vi "nanocal -- nuclear schottky fit -- 2x2 -- V9.vi"() -> ()   [LabVIEW 2021] (continued)
τ1\" -> 0.000000000000   ,  \"τS\" -> 0.000000000000   ,  \"τN\" -> 0.000000000000   ,  \"τC\" -> 0.000000000000   ,  \"κ0\" -> 0.000000000000   ,  \"mm1\" -> 0.000000000000   ,  \"mm2\" -> 0.000000000000   ,  \"mm3\" -> 0.000000000000   ,  \"T\" -> 0.300000000000   ,  \"B\" -> 10.000000000000   ,  \"θ\" -> 90.000000000000   ,  \"Reoff\" -> 0.000000000000   ,  \"Imoff\" -> 0.000000000000   ,  \"στ1\" -> 0.000000000000   ,  \"στS\" -> 0.000000000000   ,  \"στN\" -> 0.000000000000    |>   , \n\"IDS0630_220611_RAW_cal__ref_\" ->   <|    \"ζ\" -> 0.079968077159   ,  \"τ1\" -> 0.028703647271   ,  \"τS\" -> 0.027787521037   ,  \"τN\" -> 0.007458471541   ,  \"τC\" -> 0.001227018439   ,  \"κ0\" -> 0.000000002002   ,  \"mm1\" -> 0.000087530349   ,  \"mm2\" -> 0.017868351082   ,  \"mm3\" -> 0.050039331111   ,  \"T\" -> 0.360000000000   ,  \"B\" -> 10.000000000000   ,  \"θ\" -> 90.000000000000   ,  \"Reoff\" -> -6897959.183673471220   ,  \"Imoff\" -> 0.000000000000   ,  \"στ1\" -> 0.003375898444   ,  \"στS\" -> 0.000219600830   ,  \"στN\" -> 0.000437287365    |>   , \n\"IDS0630_220611_RAW_cal__sam_\" ->   <|    \"ζ\" -> 0.000000000000   ,  \"τ1\" -> 0.000000000000   ,  \"τS\" -> 0.000000000000   ,  \"τN\" -> 0.000000000000   ,  \"τC\" -> 0.000000000000   ,  \"κ0\" -> 0.000000000000   ,  \"mm1\" -> 0.000000000000   ,  \"mm2\" -> 0.000000000000   ,  \"mm3\" -> 0.000000000000   ,  \"T\" -> 0.360000000000   ,  \"B\" -> 10.000000000000   ,  \"θ\" -> 90.000000000000   ,  \"Reoff\" -> 0.000000000000   ,  \"Imoff\" -> 0.000000000000   ,  \"στ1\" -> 0.000000000000   ,  \"στS\" -> 0.000000000000   ,  \"στN\" -> 0.000000000000    |>   , \n\"IDS0631_220611_RAW_cal__ref_\" ->   <|    \"ζ\" -> 0.058778460979   ,  \"τ1\" -> 0.022115004364   ,  \"τS\" -> 0.025871969436   ,  \"τN\" -> 0.004788101555   ,  \"τC\" -> 0.001625064800   ,  \"κ0\" -> 0.000000002412   ,  \"mm1\" -> 0.000085411879   ,  \"mm2\" -> 0.015917070637   ,  \"mm3\" -> 0.040199809426   ,  \"T\" -> 0.420000000000   ,  \"B\" -> 10.000000000000   ,  \"θ\" -> 90.000000000000   ,  \"Reoff\" -> -2816326.530612244270   ,  \"Imoff\" -> 0.000000000000   ,  \"στ1\" -> 0.000587796710   ,  \"στS\" -> 0.000091605589   ,  \"στN\" -> 0.000126012019    |>   , \n\"IDS0631_220611_RAW_cal__sam_\" ->   <|    \"ζ\" -> 0.000000000000   ,  \"τ1\" -> 0.000000000000   ,  \"τS\" -> 0.000000000000   ,  \"τN\" -> 0.000000000000   ,  \"τC\" -> 0.000000000000   ,  \"κ0\" -> 0.000000000000   ,  \"mm1\" -> 0.000000000000   ,  \"mm2\" -> 0.000000000000   ,  \"mm3\" -> 0.000000000000   ,  \"T\" -> 0.420000000000   ,  \"B\" -> 10.000000000000   ,  \"θ\" -> 90.000000000000   ,  \"Reoff\" -> 0.000000000000   ,  \"Imoff\" -> 0.000000000000   ,  \"στ1\" -> 0.000000000000   ,  \"στS\" -> 0.000000000000   ,  \"στN\" -> 0.000000000000    |>   , \n\"IDS0632_220611_RAW_cal__ref_\" ->   <|    \"ζ\" -> 0.043876208110   ,  \"τ1\" -> 0.021478355659   ,  \"τS\" -> 0.024271049020   ,  \"τN\" -> 0.002270431826   ,  \"τC\" -> 0.001878964186   ,  \"κ0\" -> 0.000000003102   ,  \"mm1\" -> 0.000073722080   ,  \"mm2\" -> 0.017307979811   ,  \"mm3\" -> 0.033681638338   ,  \"T\" -> 0.520000000000   ,  \"B\" -> 10.000000000000   ,  \"θ\" -> 90.000000000000   ,  \"Reoff\" -> -1918367.346938774920   ,  \"Imoff\" -> 0.000000000000   ,  \"στ1\" -> 0.003137180042   ,  \"στS\" -> 0.000114620716   ,  \"στN\" -> 0.000177904413    |>   , \n\"IDS0632_220611_RAW_cal__sam_\" ->   <|    \"ζ\" -> 0.000000000000   ,  \"τ1\" -> 0.000000000000   ,  \"τS\" -> 0.000000000000   ,  \"τN\" -> 0.000000000000   ,  \"τC\" -> 0.000000000000   ,  \"κ0\" -> 0.000000000000   ,  \"mm1\" -> 0.000000000000   ,  \"mm2\" -> 0.000000000000   ,  \"mm3\" -> 0.000000000000   ,  \"T\" -> 0.520000000000   ,  \"B\" -> 10.000000000000   ,  \"θ\" -> 90.000000000000   ,  \"Reoff\" -> 0.000000000000   ,  \"Imoff\" -> 0.000000000000   ,  \"στ1\" -> 0.000000000000   ,  \"στS\" -> 0.000000000000   ,  \"στN\" -> 0.000000000000    |>   , \n\"IDS0633_220611_RAW_cal__ref_\" ->   <|    \"ζ\" -> 0.034677079160   ,  \"τ1\" -> 0.021718381386   ,  \"τS\" -> 0.023156430325   ,  \"τN\" -> 0.001263823282   ,  \"τC\" -> 0.002065959541   ,  \"κ0\" -> 0.000000003789   ,  \"mm1\" -> 0.000063900017   ,  \"mm2\" -> 0.018485786163   ,  \"mm3\" -> 0.030501731422   ,  \"T\" -> 0.620000000000   ,  \"B\" -> 10.000000000000   ,  \"θ\" -> 90.000000000000   ,  \"Reoff\" -> -1265306.122448978950   ,  \"Imoff\" -> 0.000000000000   ,  \"στ1\" -> 0.002060583109   ,  \"στS\" -> 0.000081647328   ,  \"στN\" -> 0.000097316031    |>   , \n\"IDS0633_220611_RAW_cal__sam_\" ->   <|    \"ζ\" -> 0.000000000000   ,  \"τ1\" -> 0.000000000000   ,  \"τS\" -> 0.000000000000   ,  \"τN\" -> 0.000000000000   ,  \"τC\" -> 0.000000000000   ,  \"κ0\" -> 0.000000000000   ,  \"mm1\" -> 0.000000000000   ,  \"mm2\" -> 0.000000000000   ,  \"mm3\" -> 0.000000000000   ,  \"T\" -> 0.620000000000   ,  \"B\" -> 10.000000000000   ,  \"θ\" -> 90.000000000000   ,  \"Reoff\" -> 0.000000000000   ,  \"Imoff\" -> 0.000000000000   ,  \"στ1\" -> 0.000000000000   ,  \"στS\" -> 0.000000000000   ,  \"στN\" -> 0.000000000000    |>   , \n\"IDS0634_220612_RAW_cal__ref_\" ->   <|    \"ζ\" -> 0.027036169383   ,  \"τ1\" -> 0.021733696350   ,  \"τS\" -> 0.021135918538   ,  \"τN\" -> 0.000553307170   ,  \"τC\" -> 0.002271656254   ,  \"κ0\" -> 0.000000005164   ,  \"mm1\" -> 0.000054257381   ,  \"mm2\" -> 0.019338329094   ,  \"mm3\" -> 0.026888385418   ,  \"T\" -> 0.820000000000   ,  \"B\" -> 10.000000000000   ,  \"θ\" -> 90.000000000000   ,  \"Reoff\" -> -938775.510204080491   ,  \"Imoff\" -> 0.000000000000   ,  \"στ1\" -> 0.001360200971   ,  \"στS\" -> 0.000123877284   ,  \"στN\" -> 0.000020166019    |>   , \n\"IDS0634_220612_RAW_cal__sam_\" ->   <|    \"ζ\" -> 0.000000000000   ,  \"τ1\" -> 0.000000000000   ,  \"τS\" -> 0.000000000000   ,  \"τN\" -> 0.000000000000   ,  \"τC\" -> 0.000000000000   ,  \"κ0\" -> 0.000000000000   ,  \"mm1\" -> 0.000000000000   ,  \"mm2\" -> 0.000000000000   ,  \"mm3\" -> 0.000000000000   ,  \"T\" -> 0.820000000000   ,  \"B\" -> 10.000000000000   ,  \"θ\" -> 90.000000000000   ,  \"Reoff\" -> 0.000000000000   ,  \"Imoff\" -> 0.000000000000   ,  \"στ1\" -> 0.000000000000   ,  \"στS\" -> 0.000000000000   ,  \"στN\" -> 0.000000000000    |>   , \n\"IDS0635_220612_RAW_cal__ref_\" ->   <|    \"ζ\" -> 0.022890647572   ,  \"τ1\" -> 0.021599440333   ,  \"τS\" -> 0.018784843036   ,  \"τN\" -> 0.000235286917   ,  \"τC\" -> 0.002353311778   ,  \"κ0\" -> 0.000000007245   ,  \"mm1\" -> 0.000047019578   ,  \"mm2\" -> 0.019399476842   ,  \"mm3\" -> 0.023961768735   ,  \"T\" -> 1.120000000000   ,  \"B\" -> 10.000000000000   ,  \"θ\" -> 90.000000000000   ,  \"Reoff\" -> -775510.204081632196   ,  \"Imoff\" -> 0.000000000000   ,  \"στ1\" -> 0.004256477992   ,  \"στS\" -> 0.000144718396   ,  \"στN\" -> 0.000029208339    |>   , \n\"IDS0635_220612_RAW_cal__sam_\" ->   <|    \"ζ\" -> 0.000000000000   ,  \"τ1\" -> 0.000000000000   ,  \"τS\" -> 0.000000000000   ,  \"τN\" -> 0.000000000000   ,  \"τC\" -> 0.000000000000   ,  \"κ0\" -> 0.000000000000   ,  \"mm1\" -> 0.000000000000   ,  \"mm2\" -> 0.000000000000   ,  \"mm3\" -> 0.000000000000   ,  \"T\" -> 1.120000000000   ,  \"B\" -> 10.000000000000   ,  \"θ\" -> 90.000000000000   ,  \"Reoff\" -> 0.000000000000   ,  \"Imoff\" -> 0.000000000000   ,  \"στ1\" -> 0.000000000000   ,  \"στS\" -> 0.000000000000   ,  \"στN\" -> 0.000000000000    |>   , \n\"IDS0636_220612_RAW_cal__ref_\" ->   <|    \"ζ\" -> 0.017457751366   ,  \"τ1\" -> 0.021556950502   ,  \"τS\" -> 0.013950093477   ,  \"τN\" -> 0.000069572481   ,  \"τC\" -> 0.002888715109   ,  \"κ0\" -> 0.000000012635   ,  \"mm1\" -> 0.000041283144   ,  \"mm2\" -> 0.016791744848   ,  \"mm3\" -> 0.021877055420   ,  \"T\" -> 1.900000000000   ,  \"B\" -> 10.000000000000   ,  \"θ\" -> 90.000000000000   ,  \"Reoff\" -> -285714.285714285448   ,  \"Imoff\" -> 0.000000000000   ,  \"στ1\" -> 0.002815711957   ,  \"στS\" -> 0.000085308545   ,  \"στN\" -> 0.000003509861    |>   , \n\"IDS0636_220612_RAW_cal__sam_\" ->   <|    \"ζ\" -> 0.000000000000   ,  \"τ1\" -> 0.000000000000   ,  \"τS\" -> 0.000000000000   ,  \"τN\" -> 0.000000000000   ,  \"τC\" -> 0.000000000000   ,  \"κ0\" -> 0.000000000000   ,  \"mm1\" -> 0.000000000000   ,  \"mm2\" -> 0.000000000000   ,  \"mm3\" -> 0.000000000000   ,  \"T\" -> 1.900000000000   ,  \"B\" -> 10.000000000000   ,  \"θ\" -> 90.000000000000   ,  \"Reoff\" -> 0.000000000000   ,  \"Imoff\" -> 0.000000000000   ,  \"στ1\" -> 0.000000000000   ,  \"στS\" -> 0.000000000000   ,  \"στN\" -> 0.000000000000    |>   , \n\"IDS0637_220612_RAW_cal__ref_\" ->   <|    \"ζ\" -> 0.017770105668   ,  \"τ1\" -> 0.021549186615   ,  \"τS\" -> 0.009965620739   ,  \"τN\" -> 0.000026194105   ,  \"τC\" -> 0.002636418134   ,  \"κ0\" -> 0.000000022540   ,  \"mm1\" -> 0.000036639875   ,  \"mm2\" -> 0.012704225708   ,  \"mm3\" -> 0.021614109615   ,  \"T\" -> 3.100000000000   ,  \"B\" -> 10.000000000000   ,  \"θ\" -> 90.000000000000   ,  \"Reoff\" -> -204081.632653061300   ,  \"Imoff\" -> 0.000000000000   ,  \"στ1\" -> 0.001593502412   ,  \"στS\" -> 0.000052874862   ,  \"στN\" -> 0.000000825186    |>   , \n\"IDS0637_220612_RAW_cal__sam_\" ->   <|    \"ζ\" -> 0.000000000000   ,  \"τ1\" -> 0.000000000000   ,  \"τS\" -> 0.000000000000   ,  \"τN\" -> 0.000000000000   ,  \"τC\" -> 0.000000000000   ,  \"κ0\" -> 0.000000000000   ,  \"mm1\" -> 0.000000000000   ,  \"mm2\" -> 0.000000000000   ,  \"mm3\" -> 0.000000000000   ,  \"T\" -> 3.100000000000   ,  \"B\" -> 10.000000000000   ,  \"θ\" -> 90.000000000000   ,  \"Reoff\" -> 0.000000000000   ,  \"Imoff\" -> 0.000000000000   ,  \"στ1\" -> 0.000000000000   ,  \"στS\" -> 0.000000000000   ,  \"στN\" -> 0.000000000000    |>   , \n\"IDS0638_220612_RAW_cal__ref_\" ->   <|    \"ζ\" -> 0.021698598791   ,  \"τ1\" -> 0.021496688345   ,  \"τS\" -> 0.006445256992   ,  \"τN\" -> 0.000009458169   ,  \"τC\" -> 0.001823286983   ,  \"κ0\" -> 0.000000055353   ,  \"mm1\" -> 0.000030436060   ,  \"mm2\" -> 0.008371803202   ,  \"mm3\" -> 0.021512509502   ,  \"T\" -> 5.700000000000   ,  \"B\" -> 10.000000000000   ,  \"θ\" -> 90.000000000000   ,  \"Reoff\" -> -122448.979591835290   ,  \"Imoff\" -> 0.000000000000   ,  \"στ1\" -> 0.002371185679   ,  \"στS\" -> 0.000866215672   ,  \"στN\" -> 0.000002921151    |>   , \n\"IDS0638_220612_RAW_cal__sam_\" ->   <|    \"ζ\" -> 0.000000000000   ,  \"τ1\" -> 0.000000000000   ,  \"τS\" -> 0.000000000000   ,  \"τN\" -> 0.000000000000   ,  \"τC\" -> 0.000000000000   ,  \"κ0\" -> 0.000000000000   ,  \"mm1\" -> 0.000000000000   ,  \"mm2\" -> 0.000000000000   ,  \"mm3\" -> 0.000000000000   ,  \"T\" -> 5.700000000000   ,  \"B\" -> 10.000000000000   ,  \"θ\" -> 90.000000000000   ,  \"Reoff\" -> 0.000000000000   ,  \"Imoff\" -> 0.000000000000   ,  \"στ1\" -> 0.000000000000   ,  \"στS\" -> 0.000000000000   ,  \"στN\" -> 0.000000000000    |>   , \n\"IDS0640_220612_RAW_cal__ref_\" ->   <|    \"ζ\" -> 0.238834044855   ,  \"τ1\" -> 0.022929416344   ,  \"τS\" -> 0.072625980306   ,  \"τN\" -> 0.019844551932   ,  \"τC\" -> 0.000823612727   ,  \"κ0\" -> 0.000000000936   ,  \"mm1\" -> 0.000157614859   ,  \"mm2\" -> 0.017180115008   ,  \"mm3\" -> 0.120970942686   ,  \"T\" -> 0.200000000000   ,  \"B\" -> 6.000000000000   ,  \"θ\" -> 90.000000000000   ,  \"Reoff\" -> -41673469.387755103400   ,  \"Imoff\" -> 0.000000000000   ,  \"στ1\" -> 0.013588787086   ,  \"στS\" -> 0.005909644069   ,  \"στN\" -> 0.005908317860    |>   , \n\"IDS0640_220612_RAW_cal__sam_\" ->   <|    \"ζ\" -> 0.000000000000   ,  \"τ1\" -> 0.000000000000   ,  \"τS\" -> 0.000000000000   ,  \"τN\" -> 0.000000000000   ,  \"τC\" -> 0.000000000000   ,  \"κ0\" -> 0.000000000000   ,  \"mm1\" -> 0.000000000000   ,  \"mm2\" -> 0.000000000000   ,  \"mm3\" -> 0.000000000000   ,  \"T\" -> 0.200000000000   ,  \"B\" -> 6.000000000000   ,  \"θ\" -> 90.000000000000   ,  \"Reoff\" -> 0.000000000000   ,  \"Imoff\" -> 0.000000000000   ,  \"στ1\" -> 0.000000000000   ,  \"στS\" -> 0.000000000000   ,  \"στN\" -> 0.000000000000    |>   , \n\"IDS0641_220612_RAW_cal__ref_\" ->   <|    \"ζ\" -> 0.337611684125   ,  \"τ1\" -> 0.024060482995   ,  \"τS\" -> 0.087442322349   ,  \"τN\" -> 0.039216913379   ,  \"τC\" -> 0.000779358096   ,  \"κ0\" -> 0.000000000742   ,  \"mm1\" -> 0.000195728848   ,  \"mm2\" -> 0.015872138171   ,  \"mm3\" -> 0.178192847684   ,  \"T\" -> 0.170000000000   ,  \"B\" -> 6.000000000000   ,  \"θ\" -> 90.000000000000   ,  \"Reoff\" -> -71142857.142857134400   ,  \"Imoff\" -> 0.000000000000   ,  \"στ1\" -> 0.018720628002   ,  \"στS\" -> 0.014050027266   ,  \"στN\" -> 0.015588773016    |>   , \n\"IDS0641_220612_RAW_cal__sam_\" ->   <|    \"ζ\" -> 0.000000000000   ,  \"τ1\" -> 0.000000000000   ,  \"τS\" -> 0.000000000000   ,  \"τN\" -> 0.000000000000   ,  \"τC\" -> 0.000000000000   ,  \"κ0\" -> 0.000000000000   ,  \"mm1\" -> 0.000000000000   ,  \"mm2\" -> 0.000000000000   ,  \"mm3\" -> 0.000000000000   ,  \"T\" -> 0.170000000000   ,  \"B\" -> 6.000000000000   ,  \"θ\" -> 90.000000000000   ,  \"Reoff\" -> 0.000000000000   ,  \"Imoff\" -> 0.000000000000   ,  \"στ1\" -> 0.000000000000   ,  \"στS\" -> 0.000000000000   ,  \"στN\" -> 0.000000000000    |>   , \n\"IDS0642_220612_RAW_cal__ref_\" ->   <|    \"ζ\" -> 0.425492131552   ,  \"τ1\" -> 0.026758245281   ,  \"τS\" -> 0.092876272141   ,  \"τN\" -> 0.068524187738   ,  \"τC\" -> 0.000712253308   ,  \"κ0\" -> 0.000000000634   ,  \"mm1\" -> 0.000211793649   ,  \"mm2\" -> 0.014653485868   ,  \"mm3\" -> 0.242680304659   ,  \"T\" -> 0.150000000000   ,  \"B\" -> 6.000000000000   ,  \"θ\" -> 90.000000000000   ,  \"Reoff\" -> -111171428.571428567000   ,  \"Imoff\" -> 0.000000000000   ,  \"στ1\" -> 0.016862211092   ,  \"στS\" -> 0.019282049224   ,  \"στN\" -> 0.022131638620    |>   , \n\"IDS0642_220612_RAW_cal__sam_\" ->   <|    \"ζ\" -> 0.000000000000   ,  \"τ1\" -> 0.000000000000   ,  \"τS\" -> 0.000000000000   ,  \"τN\" -> 0.000000000000   ,  \"τC\" -> 0.000000000000   ,  \"κ0\" -> 0.000000000000   ,  \"mm1\" -> 0.000000000000   ,  \"mm2\" -> 0.000000000000   ,  \"mm3\" -> 0.000000000000   ,  \"T\" -> 0.150000000000   ,  \"B\" -> 6.000000000000   ,  \"θ\" -> 90.000000000000   ,  \"Reoff\" -> 0.000000000000   ,  \"Imoff\" -> 0.000000000000   ,  \"στ1\" -> 0.000000000000   ,  \"στS\" -> 0.000000000000   ,  \"στN\" -> 0.000000000000    |>   , \n\"IDS0643_220612_RAW_cal__ref_\" ->   <|    \"ζ\" -> 0.645665826507   ,  \"τ1\" -> 0.033591555956   ,  \"τS\" -> 0.115598019979   ,  \"τN\" -> 0.189817561833   ,  \"τC\" -> 0.000794602780   ,  \"κ0\" -> 0.000000000472   ,  \"mm1\" -> 0.000310954135   ,  \"mm2\" -> 0.012215752320   ,  \"mm3\" -> 0.524471438152   ,  \"T\" -> 0.120000000000   ,  \"B\" -> 6.000000000000   ,  \"θ\" -> 90.000000000000   ,  \"Reoff\" -> -174187755.102040827000   ,  \"Imoff\" -> 0.000000000000   ,  \"στ1\" -> 0.039640874529   ,  \"στS\" -> 0.065981071320   ,  \"στN\" -> 0.095740947662    |>   , \n\"IDS0643_220612_RAW_cal__sam_\" ->   <|    \"ζ\" -> 0.000000000000   ,  \"τ1\" -> 0.000000000000   ,  \"τS\" -> 0.000000000000   ,  \"τN\" -> 0.000000000000   ,  \"τC\" -> 0.000000000000   ,  \"κ0\" -> 0.000000000000   ,  \"mm1\" -> 0.000000000000   ,  \"mm2\" -> 0.000000000000   ,  \"mm3\" -> 0.000000000000   ,  \"T\" -> 0.120000000000   ,  \"B\" -> 6.000000000000   ,  \"θ\" -> 90.000000000000   ,  \"Reoff\" -> 0.000000000000   ,  \"Imoff\" -> 0.000000000000   ,  \"στ1\" -> 0.000000000000   ,  \"στS\" -> 0.000000000000   ,  \"στN\" -> 0.000000000000    |>   , \n\"IDS0644_220612_RAW_cal__ref_\" ->   <|    \"ζ\" -> 0.159858410781   ,  \"τ1\" -> 0.020749494118   ,  \"τS\" -> 0.057576161881   ,  \"τN\" -> 0.009325169153   ,  \"τC\" -> 0.000895206146   ,  \"κ0\" -> 0.000000001246   ,  \"mm1\" -> 0.000121968889   ,  \"mm2\" -> 0.017087577763   ,  \"mm3\" -> 0.082031225104   ,  \"T\" -> 0.250000000000   ,  \"B\" -> 6.000000000000   ,  \"θ\" -> 90.000000000000   ,  \"Reoff\" -> -22730612.244897957900   ,  \"Imoff\" -> 0.000000000000   ,  \"στ1\" -> 0.009289428349   ,  \"στS\" -> 0.001695199729   ,  \"στN\" -> 0.001606279892    |>   , \n\"IDS0644_220612_RAW_cal__sam_\" ->   <|    \"ζ\" -> 0.000000000000   ,  \"τ1\" -> 0.000000000000   ,  \"τS\" -> 0.000000000000   ,  \"τN\" -> 0.000000000000   ,  \"τC\" -> 0.000000000000   ,  \"κ0\" -> 0.000000000000   ,  \"mm1\" -> 0.000000000000   ,  \"mm2\" -> 0.000000000000   ,  \"mm3\" -> 0.000000000000   ,  \"T\" -> 0.250000000000   ,  \"B\" -> 6.000000000000   ,  \"θ\" -> 90.000000000000   ,  \"Reoff\" -> 0.000000000000   ,  \"Imoff\" -> 0.000000000000   ,  \"στ1\" -> 0.000000000000   ,  \"στS\" -> 0.000000000000   ,  \"στN\" -> 0.000000000000    |>   , \n\"IDS0645_220612_RAW_cal__ref_\" ->   <|    \"ζ\" -> 0.118910946323   ,  \"τ1\" -> 0.019234304410   ,  \"τS\" -> 0.048411086474   ,  \"τN\" -> 0.005189783920   ,  \"τC\" -> 0.000853285420   ,  \"κ0\" -> 0.000000001572   ,  \"mm1\" -> 0.000089420282   ,  \"mm2\" -> 0.016698334707   ,  \"mm3\" -> 0.063274435457   ,  \"T\" -> 0.300000000000   ,  \"B\" -> 6.000000000000   ,  \"θ\" -> 90.000000000000   ,  \"Reoff\" -> -17734693.877551019200   ,  \"Imoff\" -> 0.000000000000   ,  \"στ1\" -> 0.002725843000   ,  \"στS\" -> 0.000632849867   ,  \"στN\" -> 0.000966939974    |>   , \n\"IDS0645_220612_RAW_cal__sam_\" ->   <|    \"ζ\" -> 0.000000000000   ,  \"τ1\" -> 0.000000000000   ,  \"τS\" -> 0.000000000000   ,  \"τN\" -> 0.000000000000   ,  \"τC\" -> 0.000000000000   ,  \"κ0\" -> 0.000000000000   ,  \"mm1\" -> 0.000000000000   ,  \"mm2\" -> 0.000000000000   ,  \"mm3\" -> 0.000000000000   ,  \"T\" -> 0.300000000000   ,  \"B\" -> 6.000000000000   ,  \"θ\" -> 90.000000000000   ,  \"Reoff\" -> 0.000000000000   ,  \"Imoff\" -> 0.000000000000   ,  \"στ1\" -> 0.000000000000   ,  \"στS\" -> 0.000000000000   ,  \"στN\" -> 0.000000000000    |>   , \n\"IDS0646_220612_RAW_cal__ref_\" ->   <|    \"ζ\" -> 0.082805615965   ,  \"τ1\" -> 0.018079378213   ,  \"τS\" -> 0.042371658617   ,  \"τN\" -> 0.002818805569   ,  \"τC\" -> 0.001126081150   ,  \"κ0\" -> 0.000000001982   ,  \"mm1\" -> 0.000084202319   ,  \"mm2\" -> 0.016434291092   ,  \"mm3\" -> 0.051619454361   ,  \"T\" -> 0.360000000000   ,  \"B\" -> 6.000000000000   ,  \"θ\" -> 90.000000000000   ,  \"Reoff\" -> -8204081.632653061300   ,  \"Imoff\" -> 0.000000000000   ,  \"στ1\" -> 0.000700707095   ,  \"στS\" -> 0.000241063025   ,  \"στN\" -> 0.000086776293    |>   , \n\"IDS0646_220612_RAW_cal__sam_\" ->   <|    \"ζ\" -> 0.000000000000   ,  \"τ1\" -> 0.000000000000   ,  \"τS\" -> 0.000000000000   ,  \"τN\" -> 0.000000000000   ,  \"τC\" -> 0.000000000000   ,  \"κ0\" -> 0.000000000000   ,  \"mm1\" -> 0.000000000000   ,  \"mm2\" -> 0.000000000000   ,  \"mm3\" -> 0.000000000000   ,  \"T\" -> 0.360000000000   ,  \"B\" -> 6.000000000000   ,  \"θ\" -> 90.000000000000   ,  \"Reoff\" -> 0.000000000000   ,  \"Imoff\" -> 0.000000000000   ,  \"στ1\" -> 0.000000000000   ,  \"στS\" -> 0.000000000000   ,  \"στN\" -> 0.000000000000    |>   , \n\"IDS0647_220612_RAW_cal__ref_\" ->   <|    \"ζ\" -> 0.061664152309   ,  \"τ1\" -> 0.016815828462   ,  \"τS\" -> 0.037558438894   ,  \"τN\" -> 0.001732753748   ,  \"τC\" -> 0.001485497584   ,  \"κ0\" -> 0.000000002383   ,  \"mm1\" -> 0.000083349881   ,  \"mm2\" -> 0.015688184969   ,  \"mm3\" -> 0.044243841925   ,  \"T\" -> 0.420000000000   ,  \"B\" -> 6.000000000000   ,  \"θ\" -> 90.000000000000   ,  \"Reoff\" -> -4297959.183673469350   ,  \"Imoff\" -> 0.000000000000   ,  \"στ1\" -> 0.001260209312   ,  \"στS\" -> 0.000277639724   ,  \"στN\" -> 0.000082943970    |>   , \n\"IDS0647_220612_RAW_cal__sam_\" ->   <|    \"ζ\" -> 0.000000000000   ,  \"τ1\" -> 0.000000000000   ,  \"τS\" -> 0.000000000000   ,  \"τN\" -> 0.000000000000   ,  \"τC\" -> 0.000000000000   ,  \"κ0\" -> 0.000000000000   ,  \"mm1\" -> 0.000000000000   ,  \"mm2\" -> 0.000000000000   ,  \"mm3\" -> 0.000000000000   ,  \"T\" -> 0.420000000000   ,  \"B\" -> 6.000000000000   ,  \"θ\" -> 90.000000000000   ,  \"Reoff\" -> 0.000000000000   ,  \"Imoff\" -> 0.000000000000   ,  \"στ1\" -> 0.000000000000   ,  \"στS\" -> 0.000000000000   ,  \"στN\" -> 0.000000000000    |>   , \n\"IDS0648_220613_RAW_cal__ref_\" ->   <|    \"ζ\" -> 0.045994195194   ,  \"τ1\" -> 0.016026096638   ,  \"τS\" -> 0.032259458883   ,  \"τN\" -> 0.001056171005   ,  \"τC\" -> 0.001611050845   ,  \"κ0\" -> 0.000000003055   ,  \"mm1\" -> 0.000067741987   ,  \"mm2\" -> 0.015191131483   ,  \"mm3\" -> 0.037226229485   ,  \"T\" -> 0.520000000000   ,  \"B\" -> 6.000000000000   ,  \"θ\" -> 90.000000000000   ,  \"Reoff\" -> -2951020.408163265330   ,  \"Imoff\" -> 0.000000000000   ,  \"στ1\" -> 0.000737061104   ,  \"στS\" -> 0.000208052023   ,  \"στN\" -> 0.000030980283    |>   , \n\"IDS0648_220613_RAW_cal__sam_\" ->   <|    \"ζ\" -> 0.000000000000   ,  \"τ1\" -> 0.000000000000   ,  \"τS\" -> 0.000000000000   ,  \"τN\" -> 0.000000000000   ,  \"τC\" -> 0.000000000000   ,  \"κ0\" -> 0.000000000000   ,  \"mm1\" -> 0.000000000000   ,  \"mm2\" -> 0.000000000000   ,  \"mm3\" -> 0.000000000000   ,  \"T\" -> 0.520000000000   ,  \"B\" -> 6.000000000000   ,  \"θ\" -> 90.000000000000   ,  \"Reoff\" -> 0.000000000000   ,  \"Imoff\" -> 0.000000000000   ,  \"στ1\" -> 0.000000000000   ,  \"στS\" -> 0.000000000000   ,  \"στN\" -> 0.000000000000    |>   , \n\"IDS0649_220613_RAW_cal__ref_\" ->   <|    \"ζ\" -> 0.039317518317   ,  \"τ1\" -> 0.015887023373   ,  \"τS\" -> 0.028743212844   ,  \"τN\" -> 0.000633963905   ,  \"τC\" -> 0.001501618583   ,  \"κ0\" -> 0.000000003740   ,  \"mm1\" -> 0.000054181024   ,  \"mm2\" -> 0.015261011828   ,  \"mm3\" -> 0.032605663538   ,  \"T\" -> 0.620000000000   ,  \"B\" -> 6.000000000000   ,  \"θ\" -> 90.000000000000   ,  \"Reoff\" -> -2861224.489795918580   ,  \"Imoff\" -> 0.000000000000   ,  \"στ1\" -> 0.000685981112   ,  \"στS\" -> 0.000220459724   ,  \"στN\" -> 0.000020766156    |>   , \n\"IDS0649_220613_RAW_cal__sam_\" ->   <|    \"ζ\" -> 0.000000000000   ,  \"τ1\" -> 0.000000000000   ,  \"τS\" -> 0.000000000000   ,  \"τN\" -> 0.000000000000   ,  \"τC\" -> 0.000000000000   ,  \"κ0\" -> 0.000000000000   ,  \"mm1\" -> 0.000000000000   ,  \"mm2\" -> 0.000000000000   ,  \"mm3\" -> 0.000000000000   ,  \"T\" -> 0.620000000000   ,  \"B\" -> 6.000000000000   ,  \"θ\" -> 90.000000000000   ,  \"Reoff\" -> 0.000000000000   ,  \"Imoff\" -> 0.000000000000   ,  \"στ1\" -> 0.000000000000   ,  \"στS\" -> 0.000000000000   ,  \"στN\" -> 0.000000000000    |>   , \n\"IDS0650_220613_RAW_cal__ref_\" ->   <|    \"ζ\" -> 0.027547170013   ,  \"τ1\" -> 0.015538067589   ,  \"τS\" -> 0.023363331371   ,  \"τN\" -> 0.000418112584   ,  \"τC\" -> 0.002109607806   ,  \"κ0\" -> 0.000000005116   ,  \"mm1\" -> 0.000052091035   ,  \"mm2\" -> 0.014959485804   ,  \"mm3\" -> 0.027072653991   ,  \"T\" -> 0.820000000000   ,  \"B\" -> 6.000000000000   ,  \"θ\" -> 90.000000000000   ,  \"Reoff\" -> -1200000.000000000000   ,  \"Imoff\" -> 0.000000000000   ,  \"στ1\" -> 0.001116730180   ,  \"στS\" -> 0.000160859553   ,  \"στN\" -> 0.000016254446    |>   , \n\"IDS0650_220613_RAW_cal__sam_\" ->   <|    \"ζ\" -> 0.000000000000   ,  \"τ1\" -> 0.000000000000   ,  \"τS\" -> 0.000000000000   ,  \"τN\" -> 0.000000000000   ,  \"τC\" -> 0.000000000000   ,  \"κ0\" -> 0.000000000000   ,  \"mm1\" -> 0.000000000000   ,  \"mm2\" -> 0.000000000000   ,  \"mm3\" -> 0.000000000000   ,  \"T\" -> 0.820000000000   ,  \"B\" -> 6.000000000000   ,  \"θ\" -> 90.000000000000   ,  \"Reoff\" -> 0.000000000000   ,  \"Imoff\" -> 0.000000000000   ,  \"στ1\" -> 0.000000000000   ,  \"στS\" -> 0.000000000000   ,  \"στN\" -> 0.000000000000    |>   , \n\"IDS0651_220613_RAW_cal__ref_\" ->   <|    \"ζ\" -> 0.024620092111   ,  \"τ1\" -> 0.015537036119   ,  \"τS\" -> 0.019312906027   ,  \"τN\" -> 0.000248247799   ,  \"τC\" -> 0.001859270827   ,  \"κ0\" -> 0.000000007154   ,  \"mm1\" -> 0.000040915639   ,  \"mm2\" -> 0.014964167926   ,  \"mm3\" -> 0.022433974616   ,  \"T\" -> 1.120000000000   ,  \"B\" -> 6.000000000000   ,  \"θ\" -> 90.000000000000   ,  \"Reoff\" -> -1200000.000000000000   ,  \"Imoff\" -> 0.000000000000   ,  \"στ1\" -> 0.002643651346   ,  \"στS\" -> 0.000176224289   ,  \"στN\" -> 0.000013219206    |>   , \n\"IDS0651_220613_RAW_cal__sam_\" ->   <|    \"ζ\" -> 0.000000000000   ,  \"τ1\" -> 0.000000000000   ,  \"τS\" -> 0.000000000000   ,  \"τN\" -> 0.000000000000   ,  \"τC\" -> 0.000000000000   ,  \"κ0\" -> 0.000000000000   ,  \"mm1\" -> 0.000000000000   ,  \"mm2\" -> 0.000000000000   ,  \"mm3\" -> 0.000000000000   ,  \"T\" -> 1.120000000000   ,  \"B\" -> 6.000000000000   ,  \"θ\" -> 90.000000000000   ,  \"Reoff\" -> 0.000000000000   ,  \"Imoff\" -> 0.000000000000   ,  \"στ1\" -> 0.000000000000   ,  \"στS\" -> 0.000000000000   ,  \"στN\" -> 0.000000000000    |>   , \n\"IDS0652_220613_RAW_cal__ref_\" ->   <|    \"ζ\" -> 0.018133168210   ,  \"τ1\" -> 0.015564889407   ,  \"τS\" -> 0.014281099211   ,  \"τN\" -> 0.000112228252   ,  \"τC\" -> 0.001668116156   ,  \"κ0\" -> 0.000000012545   ,  \"mm1\" -> 0.000026695788   ,  \"mm2\" -> 0.014547678858   ,  \"mm3\" -> 0.017312955008   ,  \"T\" -> 1.900000000000   ,  \"B\" -> 6.000000000000   ,  \"θ\" -> 90.000000000000   ,  \"Reoff\" -> -571428.571428570895   ,  \"Imoff\" -> 0.000000000000   ,  \"στ1\" -> 0.001046681870   ,  \"στS\" -> 0.000127218281   ,  \"στN\" -> 0.000003793183    |>   , \n\"IDS0652_220613_RAW_cal__sam_\" ->   <|    \"ζ\" -> 0.000000000000   ,  \"τ1\" -> 0.000000000000   ,  \"τS\" -> 0.000000000000   ,  \"τN\" -> 0.000000000000   ,  \"τC\" -> 0.000000000000   ,  \"κ0\" -> 0.000000000000   ,  \"mm1\" -> 0.000000000000   ,  \"mm2\" -> 0.000000000000   ,  \"mm3\" -> 0.000000000000   ,  \"T\" -> 1.900000000000   ,  \"B\" -> 6.000000000000   ,  \"θ\" -> 90.000000000000   ,  \"Reoff\" -> 0.000000000000   ,  \"Imoff\" -> 0.000000000000   ,  \"στ1\" -> 0.000000000000   ,  \"στS\" -> 0.000000000000   ,  \"στN\" -> 0.000000000000    |>   , \n\"IDS0653_220613_RAW_cal__ref_\" ->   <|    \"ζ\" -> 0.015908509188   ,  \"τ1\" -> 0.015560123784   ,  \"τS\" -> 0.010437245612   ,  \"τN\" -> 0.000039412596   ,  \"τC\" -> 0.001682576218   ,  \"κ0\" -> 0.000000022391   ,  \"mm1\" -> 0.000022781914   ,  \"mm2\" -> 0.012121954903   ,  \"mm3\" -> 0.015741289406   ,  \"T\" -> 3.100000000000   ,  \"B\" -> 6.000000000000   ,  \"θ\" -> 90.000000000000   ,  \"Reoff\" -> -257142.857142856344   ,  \"Imoff\" -> 0.000000000000   ,  \"στ1\" -> 0.001376449847   ,  \"στS\" -> 0.000104641976   ,  \"στN\" -> 0.000001510582    |>   , \n\"IDS0653_220613_RAW_cal__sam_\" ->   <|    \"ζ\" -> 0.000000000000   ,  \"τ1\" -> 0.000000000000   ,  \"τS\" -> 0.000000000000   ,  \"τN\" -> 0.000000000000   ,  \"τC\" -> 0.000000000000   ,  \"κ0\" -> 0.000000000000   ,  \"mm1\" -> 0.000000000000   ,  \"mm2\" -> 0.000000000000   ,  \"mm3\" -> 0.000000000000   ,  \"T\" -> 3.100000000000   ,  \"B\" -> 6.000000000000   ,  \"θ\" -> 90.000000000000   ,  \"Reoff\" -> 0.000000000000   ,  \"Imoff\" -> 0.000000000000   ,  \"στ1\" -> 0.000000000000   ,  \"στS\" -> 0.000000000000   ,  \"στN\" -> 0.000000000000    |>   , \n\"IDS0654_220613_RAW_cal__ref_\" ->   <|    \"ζ\" -> 0.019038104176   ,  \"τ1\" -> 0.015490030186   ,  \"τS\" -> 0.006638290269   ,  \"τN\" -> 0.000014977191   ,  \"τC\" -> 0.001402127213   ,  \"κ0\" -> 0.000000055099   ,  \"mm1\" -> 0.000021755736   ,  \"mm2\" -> 0.008128200279   ,  \"mm3\" -> 0.015522134442   ,  \"T\" -> 5.700000000000   ,  \"B\" -> 6.000000000000   ,  \"θ\" -> 90.000000000000   ,  \"Reoff\" -> -122448.979591837153   ,  \"Imoff\" -> 0.000000000000   ,  \"στ1\" -> 0.001473863234   ,  \"στS\" -> 0.001201981079   ,  \"στN\" -> 0.000006042415    |>   , \n\"IDS0654_220613_RAW_cal__sam_\" ->   <|    \"ζ\" -> 0.000000000000   ,  \"τ1\" -> 0.000000000000   ,  \"τS\" -> 0.000000000000   ,  \"τN\" -> 0.000000000000   ,  \"τC\" -> 0.000000000000   ,  \"κ0\" -> 0.000000000000   ,  \"mm1\" -> 0.000000000000   ,  \"mm2\" -> 0.000000000000   ,  \"mm3\" -> 0.000000000000   ,  \"T\" -> 5.700000000000   ,  \"B\" -> 6.000000000000   ,  \"θ\" -> 90.000000000000   ,  \"Reoff\" -> 0.000000000000   ,  \"Imoff\" -> 0.000000000000   ,  \"στ1\" -> 0.000000000000   ,  \"στS\" -> 0.000000000000   ,  \"στN\" -> 0.000000000000    |>   , \n\"IDS0656_220614_RAW_cal__ref_\" ->   <|    \"ζ\" -> 0.114980929436   ,  \"τ1\" -> 0.032962817250   ,  \"τS\" -> 0.035017096889   ,  \"τN\" -> 0.003080741681   ,  \"τC\" -> 0.000981599514   ,  \"κ0\" -> 0.000000001554   ,  \"mm1\" -> 0.000098987844   ,  \"mm2\" -> 0.026319221662   ,  \"mm3\" -> 0.050004570716   ,  \"T\" -> 0.300000000000   ,  \"B\" -> 4.000000000000   ,  \"θ\" -> 90.000000000000   ,  \"Reoff\" -> -14408163.265306145000   ,  \"Imoff\" -> 0.000000000000   ,  \"στ1\" -> 0.004085076659   ,  \"στS\" -> 0.000415897428   ,  \"στN\" -> 0.000257564031    |>   , \n\"IDS0656_220614_RAW_cal__sam_\" ->   <|    \"ζ\" -> 0.000000000000   ,  \"τ1\" -> 0.000000000000   ,  \"τS\" -> 0.000000000000   ,  \"τN\" -> 0.000000000000   ,  \"τC\" -> 0.000000000000   ,  \"κ0\" -> 0.000000000000   ,  \"mm1\" -> 0.000000000000   ,  \"mm2\" -> 0.000000000000   ,  \"mm3\" -> 0.000000000000   ,  \"T\" -> 0.300000000000   ,  \"B\" -> 4.000000000000   ,  \"θ\" -> 90.000000000000   ,  \"Reoff\" -> 0.000000000000   ,  \"Imoff\" -> 0.000000000000   ,  \"στ1\" -> 0.000000000000   ,  \"στS\" -> 0.000000000000   ,  \"στN\" -> 0.000000000000    |>   , \n"
  in  "cspan":dbl=0.02 format="%#_13g"
  in  "landscape plots":enum32{"Page 1", "Page 2"}(tab)
  in  "range one":dbl(slide)=0.006965 min=0.0 max=0.3 step=1e-06 scale=0.0001..1.0 scale format="%#_3p"
  in  "one":T2=enum."τS"
  out "Plot: goodness":cluster{"Freq out (Hz)":dbl[], dbl[]}[](graph)
  in  "plot landscape!":bool
  in  "range two":dbl(slide)=0.0039049999999999996 min=0.0 max=0.3 step=1e-06 scale=0.0001..1.0 scale format="%#_3p"
  in  "two":T2=enum."τ1"
  in  "what":enum16{"1d plots", "2d plots "}(ring)
  in  "# points":i32=200
  in  "Array":T2[](array[typedef])=[enum."ζ", enum."τ1", enum."τS", enum."τN", enum."τC"]
  in  "color Map":map{T2, u32}(c390)
